vi "X Y to Angle.vi"(2 "y":dbl, 3 "x":dbl) -> (0 "Heading Out (deg)":dbl, 1 "Heading Out (rad)":dbl)   [LabVIEW 2011]
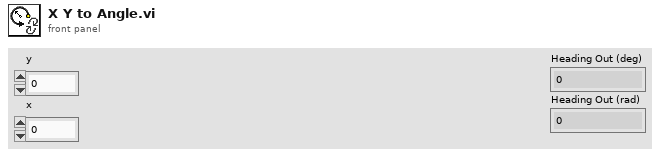
[diagram p1: front panel]
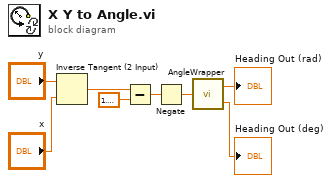
[diagram p0: block diagram]
diagram:
  n1 = Inverse Tangent (2 Input)(1:"x", 2:"y") -> (0:w6:dbl)
  n2 = Subtract(x=w6, y=1.5707963267948966) -> (x-y=w4:dbl)
  n3 = Negate(x=w4) -> (-x=w3:dbl)
  n4 = call "AngleWrapper.vi"("Heading In (rad)"=w3) -> ("Heading Out (rad)"=→"Heading Out (rad)":dbl, "Heading Out (deg)"=→"Heading Out (deg)":dbl)
